vi "XIPIN_DisplayPort_TX_Subsystem_1_0.vi"   [LabVIEW 2017]
doc: "The DisplayPort TX Subsystem connects one or more AXI4-Stream interfaces to DisplayPort\n------------------------------------\n<b>Need License</b> : Yes\n<b>Interface</b> : AXI4 AXI4-Stream"
uses:
  <vilib>/rvi/XilinxIP/XIPIN_XNode/niFpgaXIPIN.xnode
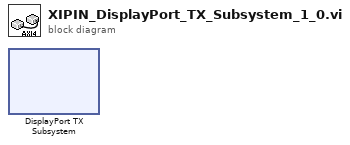
[diagram p0: block diagram]
diagram:
  n1 = xnode ("DisplayPort TX Subsystem")() -> ()
